vi "Read.vi"(6 "Append Index":i32, 8 "error in (no error)":errorcluster, 11 "Data Save in":refnum<class "Data.lvclass">) -> (0 "error out":errorcluster, 1 "Notes":string, 2 "Data (Dictionary)":T1[](array[typedef]), 3 "Data Save out":refnum<class "Data.lvclass">, 5 "Path out":path)   [LabVIEW 2019, in "Data.lvclass"]
uses:
  Data.lvclass
  Typedefs/Dictionary--cluster.ctl
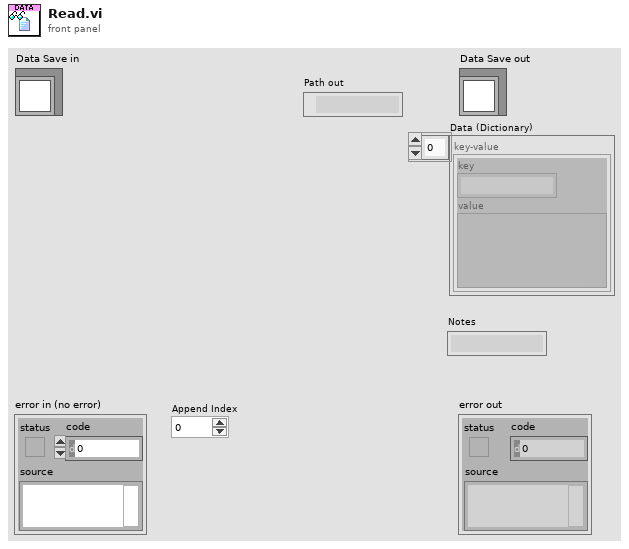
[diagram p1: front panel]
types:
  T1 = typedef "Data.lvclass/Dictionary--cluster.ctl" = cluster{"key":string, "value":variant}
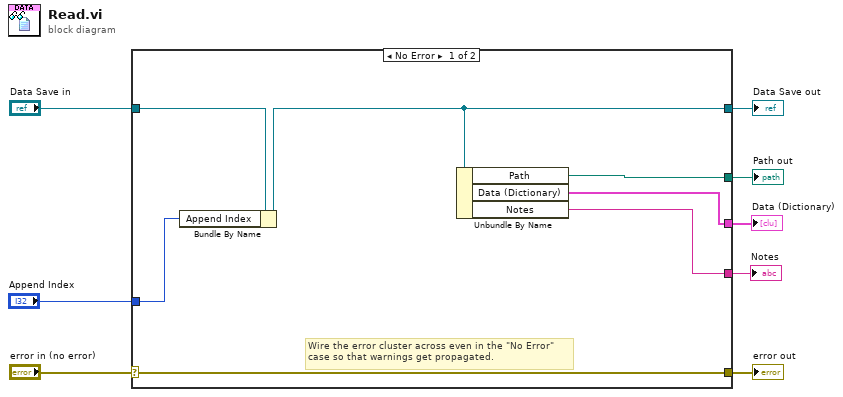
[diagram p0: block diagram]
diagram:
  n1 = case shown="No Error" "error in (no error)" {
    selector: "error in (no error)" -> [w15 w17]
    tunnel: [w15 w17] -> w7
    tunnel: [w10 w16] -> w5
    tunnel: "Data Save in" -> [w11 w16]
    tunnel: [w14 _] -> w4
    tunnel: [w13 _] -> w3
    tunnel: [w12 _] -> w2
    tunnel: "Append Index" -> [w9 _]
    frame No Error {
      # "Wire the error cluster across even in the \"No Error\"\ncase so that warnings get propagated."
      n2 = Bundle By Name(cluster=w11, "Append Index"=w9) -> (w10:refnum<class "Data.lvclass">)
      n3 = Unbundle By Name(w10) -> ("Path"=w14:path, "Data (Dictionary)"=w13:T1[], "Notes"=w12:string)
    }
    frame Error {
    }
  }
  "error out" <- w7
  "Data Save out" <- w5
  "Path out" <- w4
  "Data (Dictionary)" <- w3
  "Notes" <- w2
